vi "Config Mods.vi"(8 "error in (no error)":errorcluster, 10 "ECAT Mod Reconfig in":T1[](array[typedef]), 11 "RSI Modules in":T2[](array[typedef]) {"Module Config Data"."Config Block Data Refs"."Data Reference" format="%.0x"; "Output Data"."Output Block Data Refs"."Data Reference" format="%.0x"; "Input Data"."Input Block Data Refs"."Data Reference" format="%.0x"; "VS ref" format="%.0x"}) -> (0 "error out":errorcluster, 2 "ECAT Mod Reconfig out":T1[](array[typedef]), 3 "RSI Modules out":T2[](array[typedef]) {"Module Config Data"."Config Block Data Refs"."Data Reference" format="%.0x"; "Output Data"."Output Block Data Refs"."Data Reference" format="%.0x"; "Input Data"."Input Block Data Refs"."Data Reference" format="%.0x"; "VS ref" format="%.0x"})   [LabVIEW 2011, in "Scan Engine Custom Device.lvlib"]
uses:
  Scan Engine Custom Device.lvlib
  Type Defs/RSI Module Data.ctl
  <vilib>/NI Veristand/Custom Device API/Custom Device Item Ref.ctl
  Modules.lvlibp/RSI Module/RSI Module.lvclass
  Modules.lvlibp/RSI Module/Module Models.ctl
  Modules.lvlibp/RSI Module/Channel Type.ctl
  Type Defs/Input Data.ctl
  <vilib>/NI Veristand/Custom Device API/Block Data Reference.ctl
  <vilib>/NI Veristand/Custom Device API/Data Reference.ctl
  Type Defs/Output Data.ctl
  Type Defs/Module Config Data.ctl
  Type Defs/Mixed IO.ctl
  Type Defs/ECAT Module Reconfig.ctl
  <vilib>/NI Veristand/Custom Device API/Custom Device API.lvlib
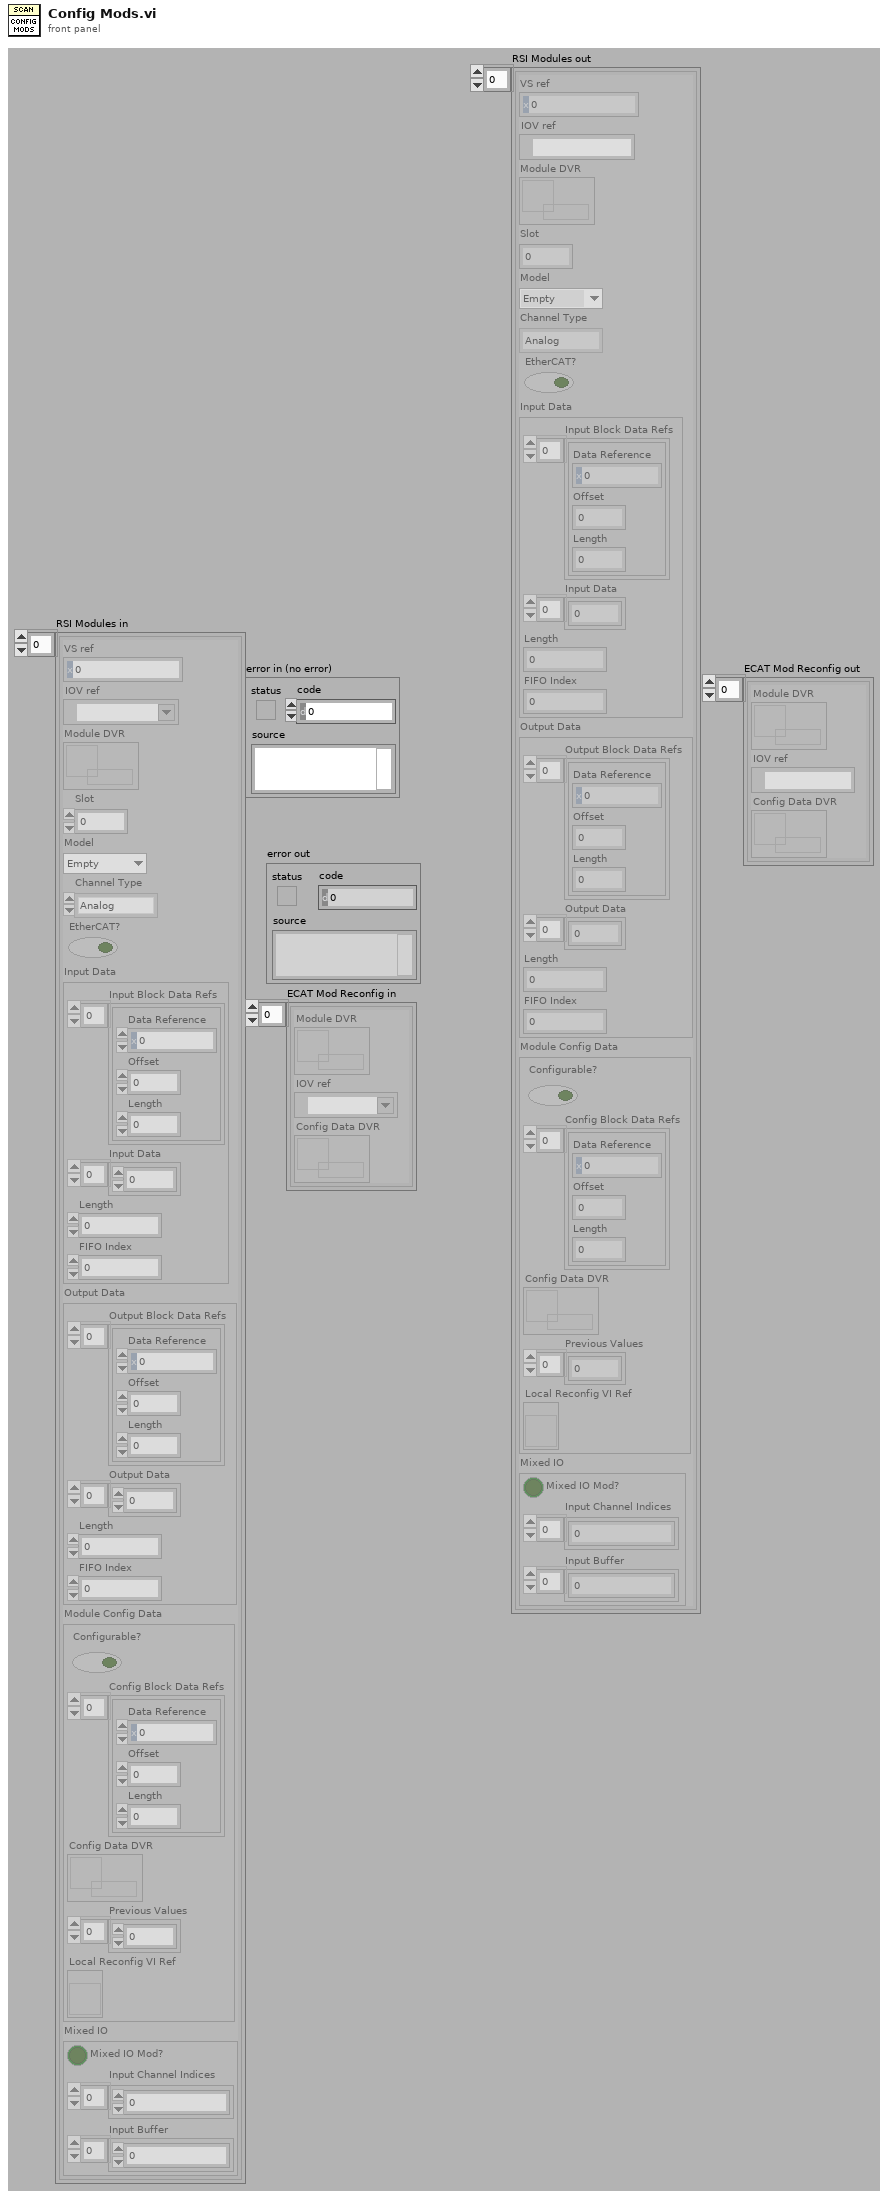
[diagram p1: front panel]
types:
  T1 = typedef "Scan Engine Custom Device.lvlib/ECAT Module Reconfig.ctl" = cluster{"Module DVR":refnum<data-value>, "IOV ref":refnum<k21>, "Config Data DVR":refnum<data-value>}
  T2 = typedef "Scan Engine Custom Device.lvlib/RSI Module Data.ctl" = cluster{"VS ref":T3, "IOV ref":refnum<k21>, "Module DVR":refnum<data-value>, "Slot":u32, "Model":T4, "Channel Type":T5, "EtherCAT?":bool, "Input Data":T6, "Output Data":T9, "Module Config Data":T10, "Mixed IO":T11}
  T3 = typedef "Custom Device API.lvlib/Custom Device Item Ref.ctl" = u64
  T4 = typedef "Modules.lvlibp/RSI Module.lvclass/Module Models.ctl" = enum16{"Empty", "NI 9201", "NI 9203", "NI 9205", "NI 9206", "NI 9207", "NI 9208", "NI 9211", "NI 9213", "NI 9214", "NI 9215", "NI 9217", "NI 9219", "NI 9221", "NI 9225", "NI 9227", "NI 9229", "NI 9233", "NI 9234", "NI 9235", "NI 9236", "NI 9237", "NI 9239", "NI 9263", "NI 9264", "NI 9265", "NI 9269", "NI 9375", "NI 9401", "NI 9402", "NI 9403", "NI 9411", "NI 9421", "NI 9422", "NI 9423", "NI 9425", "NI 9426", "NI 9435", "NI 9472", "NI 9474", "NI 9475", "NI 9476", "NI 9477", "NI 9478", "NI 9481", "NI 9482", "NI 9485"}
  T5 = typedef "Modules.lvlibp/RSI Module.lvclass/Channel Type.ctl" = enum16{"Analog", "Digital"}
  T6 = typedef "Scan Engine Custom Device.lvlib/Input Data.ctl" = cluster{"Input Block Data Refs":T7[], "Input Data":dbl[], "Length":i32, "FIFO Index":i32}
  T7 = typedef "Custom Device API.lvlib/Block Data Reference.ctl" = cluster{"Data Reference":T8, "Offset":i32, "Length":i32}
  T8 = typedef "Custom Device API.lvlib/Data Reference.ctl" = i32
  T9 = typedef "Scan Engine Custom Device.lvlib/Output Data.ctl" = cluster{"Output Block Data Refs":T7[], "Output Data":dbl[], "Length":i32, "FIFO Index":i32}
  T10 = typedef "Scan Engine Custom Device.lvlib/Module Config Data.ctl" = cluster{"Configurable?":bool, "Config Block Data Refs":T7[], "Config Data DVR":refnum<data-value>, "Previous Values":dbl[], "Local Reconfig VI Ref":refnum<vi>}
  T11 = typedef "Scan Engine Custom Device.lvlib/Mixed IO.ctl" = cluster{"Mixed IO Mod?":bool, "Input Channel Indices":i32[], "Input Buffer":dbl[]}
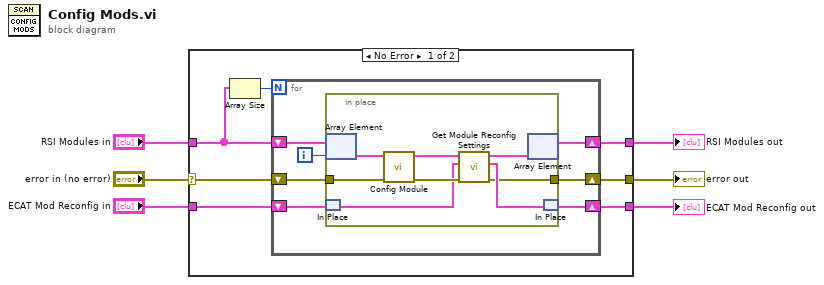
[diagram p0: block diagram]
diagram:
  n1 = case shown="No Error" "error in (no error)" {
    selector: "error in (no error)" -> [w7 w31]
    tunnel: "RSI Modules in" -> [w12 w30]
    tunnel: [w11 w30] -> w5
    tunnel: [w10 w31] -> w4
    tunnel: "ECAT Mod Reconfig in" -> [w9 w29]
    tunnel: [w8 w29] -> w2
    frame No Error {
      n2 = Array Size(array=w12) -> (size(s)=w13:i32)
      n3 = for {
        N: w13 -> [_]
        shift-right: [w16] -> w10
        shift-left: w7 -> [w18]
        shift-right: [w17] -> w11
        shift-left: w12 -> [w20]
        shift-right: [w14] -> w8
        shift-left: w9 -> [w15]
        i -> [w19]
        n4 = in-place {
          in-place-border: w18 -> [w27]
          in-place-border: [w21] -> w16
          n5 = in-place-array #1(w20, w19) -> (w28:T2)
          n6 = in-place-match #2(w15) -> (w24:T1[])
          n7 = call "Config Module.vi"("error in (no error)"=w27, "RSI Module in"=w28) -> ("error out"=w25:errorcluster, "RSI Module out"=w26:T2)  [unwired: 8 in]
          n8 = call "Get Module Reconfig Settings.vi"("error in (no error)"=w25, "ECAT Mod Reconfig in"=w24, "RSI Module in"=w26) -> ("error out"=w21:errorcluster, "ECAT Mod Reconfig out"=w23:T1[], "RSI Module out"=w22:T2)  [unwired: 6 in]
          n9 = in-place-array #1(w22) -> (w17:T2[])  [unwired: 1 out]
          n10 = in-place-match #2(w23) -> (w14:T1[])
        }
      }
    }
    frame Error {
    }
  }
  "RSI Modules out" <- w5
  "error out" <- w4
  "ECAT Mod Reconfig out" <- w2
